vi "Acquire.vi"(8 "error in (no error)":errorcluster, 10 "Digital Write Status":bool[][](array[boolean]), 11 "Hardware Resources in":T1) -> (0 "error out":errorcluster, 2 "data":waveform(dbl)[](array[waveform]), 3 "Hardware Resources out":T1)   [LabVIEW 2018, in "DAQ.lvlib"]
doc: "Perform the acquisition. Replace the contents of this diagram with calls to acquisition hardware."
uses:
  DAQ/DAQ.lvlib
  Hardware Configuration.ctl
  Task Cluster.ctl
  <vilib>/DAQmx/read.llb/DAQmx Read (Analog 1D Wfm NChan NSamp).vi
  <vilib>/DAQmx/write.llb/DAQmx Write (Digital 1D Bool NChan 1Samp 1Line).vi
  <vilib>/DAQmx/miscellaneous.llb/DAQmx Fill In Error Info.vi
  <resource>/objmgr/daqmx.rc
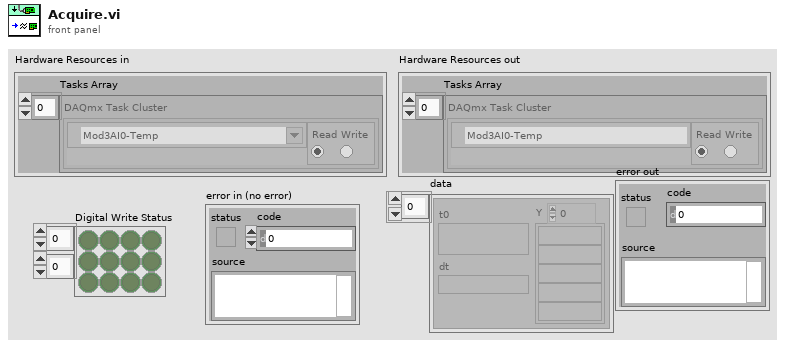
[diagram p1: front panel]
types:
  T1 = typedef "DAQ.lvlib/Hardware Configuration.ctl" = cluster{"Tasks Array":T2[]}
  T2 = typedef "Task Cluster.ctl" = cluster{"DAQmx Task":refnum<k21>, "Read-Write Radio":enum32{"Read", "Write"}}
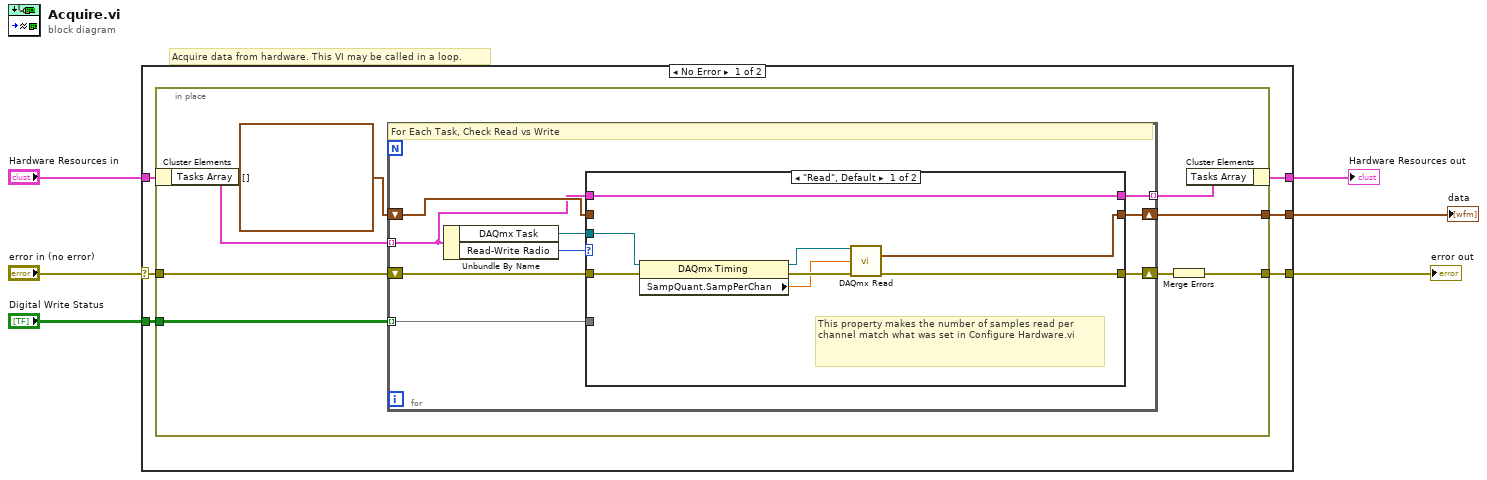
[diagram p0: block diagram]
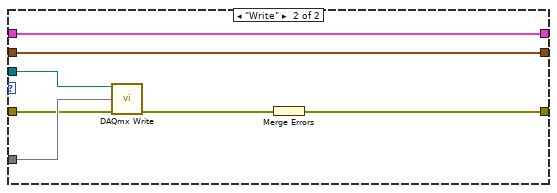
[diagram p2: hidden frame]
diagram:
  # "Acquire data from hardware. This VI may be called in a loop."
  n1 = case shown="No Error" "error in (no error)" {
    selector: "error in (no error)" -> [w11 w45]
    tunnel: [w12 w45] -> w5
    tunnel: "Hardware Resources in" -> [w8 w46]
    tunnel: [w7 w46] -> w3
    tunnel: [w9 _] -> w2
    tunnel: "Digital Write Status" -> [w10 _]
    frame No Error {
      n2 = in-place {
        in-place-border: [w20] -> w12
        in-place-border: w11 -> [w18]
        in-place-border: w10 -> [w17]
        in-place-border: [w16] -> w9
        n3 = in-place-cluster #1(w8) -> ("Tasks Array"=w14:T2[])
        n4 = for {
          tunnel: w14 -> [w22] mode=indexing
          shift-right: [w24] -> w19
          shift-left: w18 -> [w29]
          tunnel: w17 -> [w25] mode=indexing
          shift-right: [w26] -> w16
          shift-left: waveform(dbl)[] [] ("data") -> [w23]
          tunnel: [w21] -> w13 mode=indexing
          # "For Each Task, Check Read vs Write"
          n5 = Unbundle By Name(w22) -> ("DAQmx Task"=w28:refnum<k21>, "Read-Write Radio"=w27:enum32{"Read", "Write"})
          n6 = case shown="\"Read\", Default" w27 {
            tunnel: [w30 w42] -> w24
            tunnel: w29 -> [w36 w41]
            tunnel: w28 -> [w33 w43]
            tunnel: [w32 w39] -> w26
            tunnel: w25 -> [_ w44]
            tunnel: w23 -> [_ w39]
            tunnel: w22 -> [w31 w38]
            tunnel: [w31 w38] -> w21
            frame "Read", Default {
              # "This property makes the number of samples read per channel match what was set in Configure Hardware.vi"
              n7 = property class="DAQmx Timing"(reference=w33, error in=w36) -> (reference out=w37:refnum<k21>, error out=w35:errorcluster, "SampQuant.SampPerChan"=w34:dbl)
              n8 = call-poly <vilib>:"DAQmx Read.vi"("task/channels in"=w37, "number of samples per channel"=w34, "error in"=w35) -> ("data"=w32:waveform(dbl)[], "error out"=w30:errorcluster)  [unwired: 10 in, 1 out]
            }
            frame "Write" {
              n9 = call-poly <vilib>:"DAQmx Write.vi"("task/channels in"=w43, "data"=w44, "error in"=w41) -> ("error out"=w40:errorcluster)  [unwired: 10 in, 2 out]
              n10 = Merge Errors(w40) -> (w42:errorcluster)
            }
          }
        }
        n11 = Merge Errors(w19) -> (w20:errorcluster)
        n12 = in-place-cluster #1("Tasks Array"=w13) -> (w7:T1)
      }
    }
    frame Error {
    }
  }
  "Hardware Resources out" <- w3
  "error out" <- w5
  "data" <- w2
